vi "MysqlTest2.vi"() -> ()   [LabVIEW 2018]
uses:
  <vilib>/addons/database/Connection.llb/DB Tools Open Connec (String).vi
  <vilib>/addons/database/NI_Database_API.lvlib
panel:
  out "连接的字符串":string
  in  "布尔":bool
  in  "主界面选项卡":enum32{"数据管理"}(tab)
  in  "查询":bool
  in  "终结时间":timestamp
  in  "起始时间":timestamp
  in  "关键字查询":string
  in  "刷新":bool
  out "当前页数":i16
  out "总页数":i16
  in  "下一页":bool
  in  "上一页":bool
  out "数据查询":string[][](table)
  out "data":string[][](table)
  out "error out":errorcluster caption="错误输出"
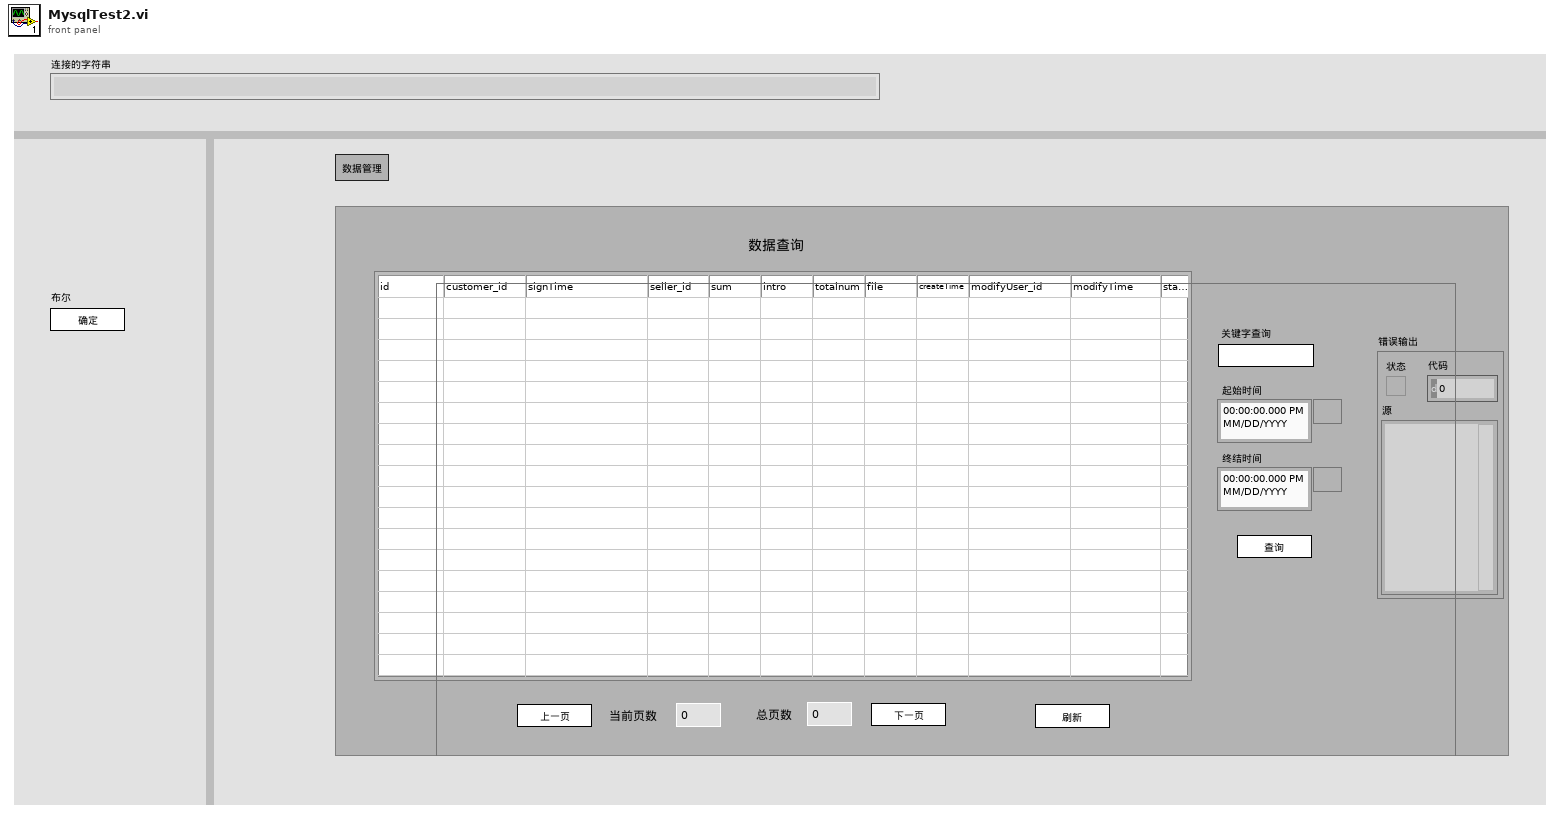
[diagram p1: front panel]
types:
  T1 = typedef "NI_Database_API.lvlib/Conn ObjectReference.ctl" = refnum<k1>
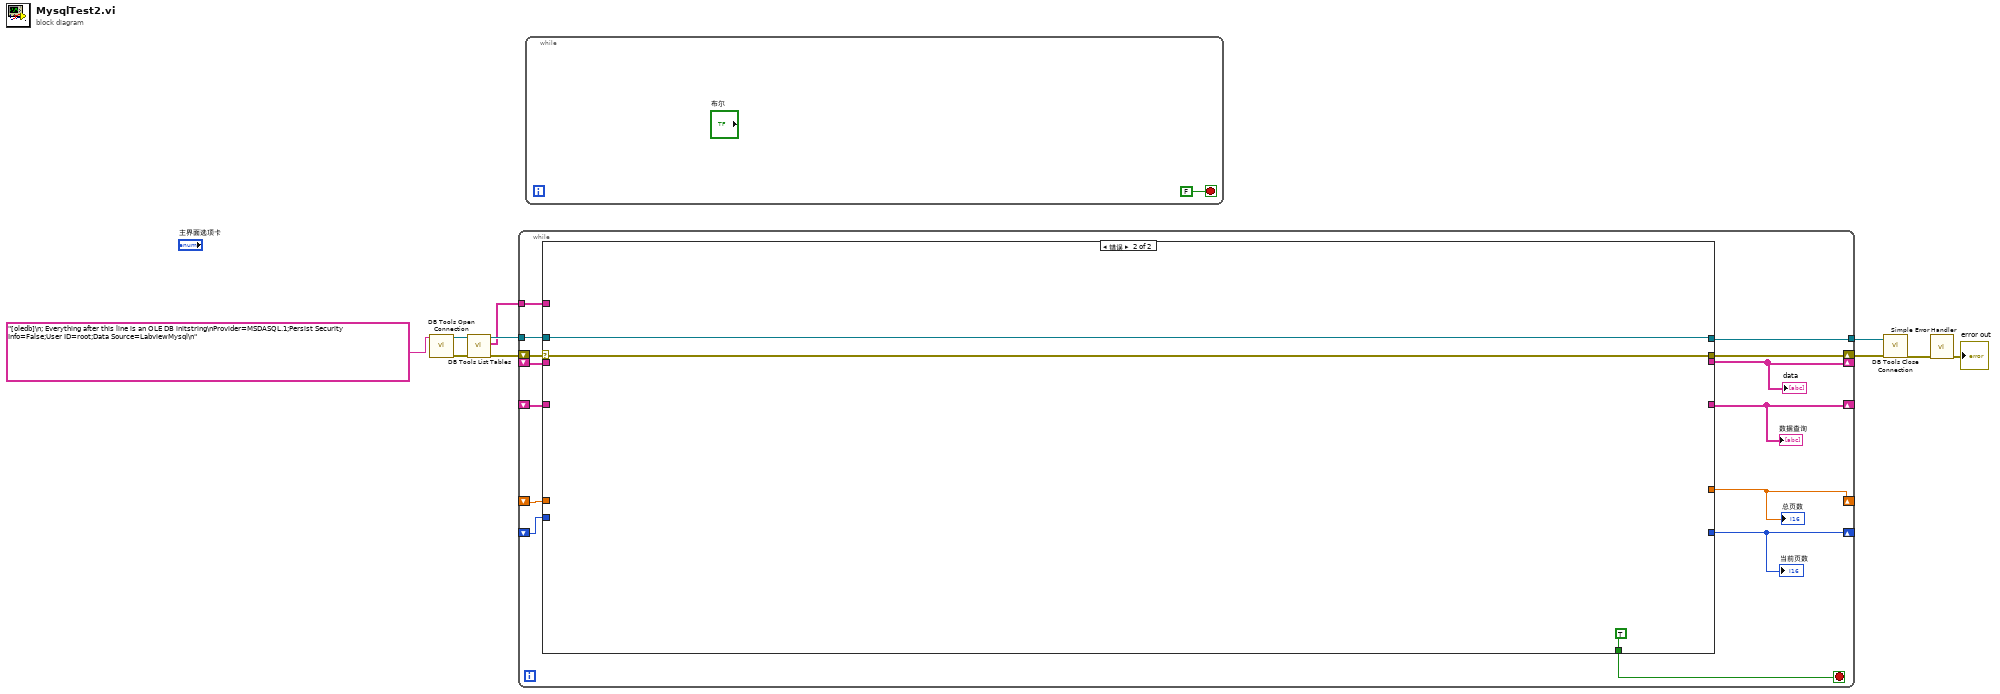
[diagram p0: block diagram]
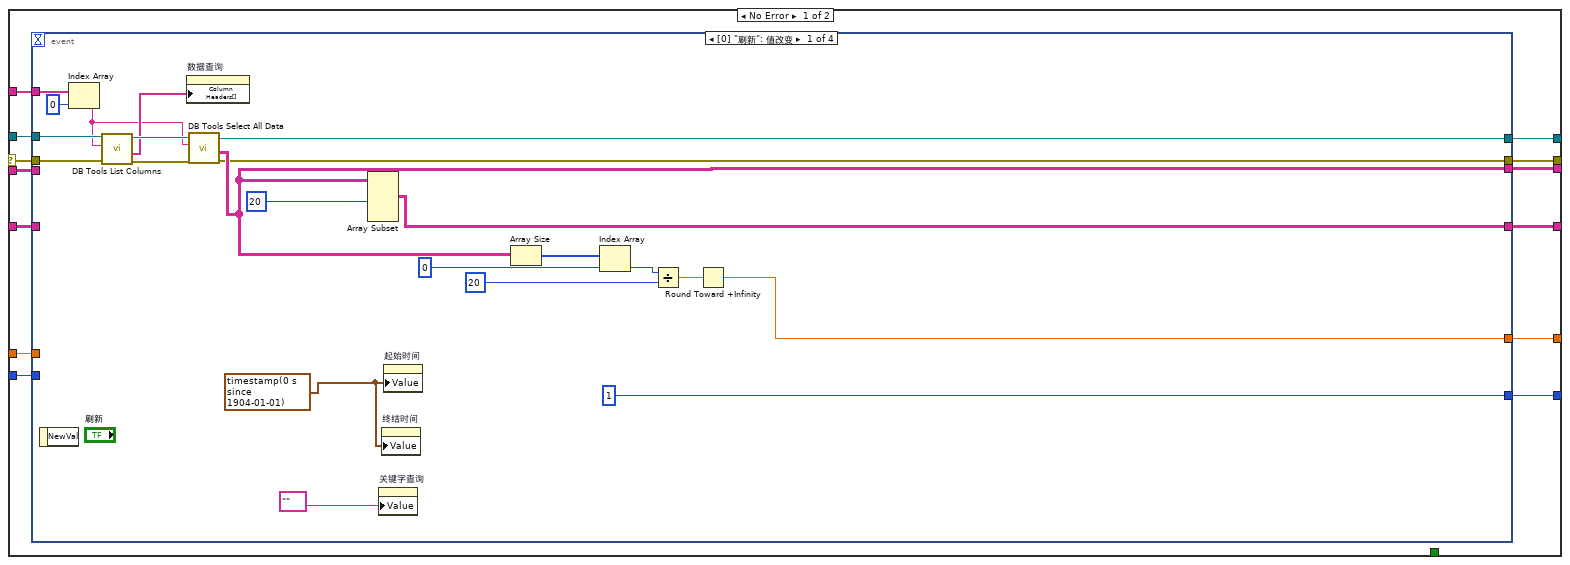
[diagram p2: hidden frame]
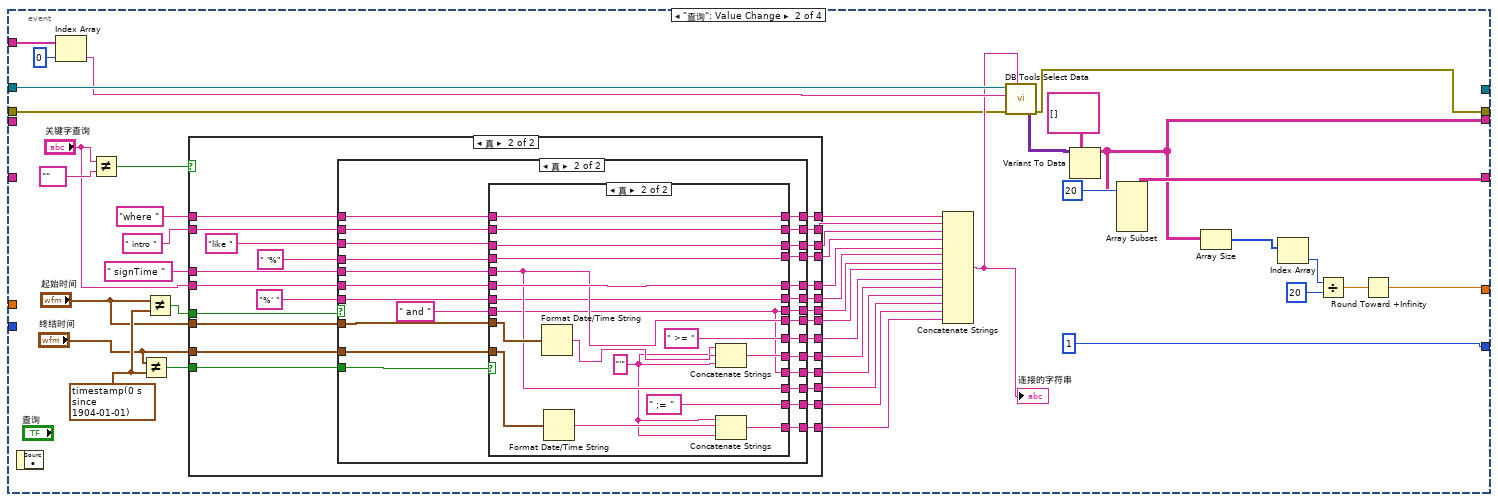
[diagram p3: hidden frame]
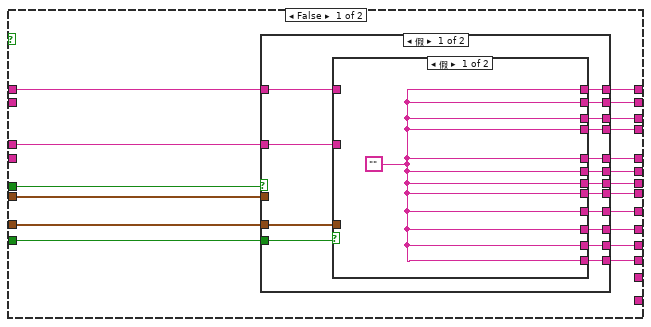
[diagram p4: hidden frame]
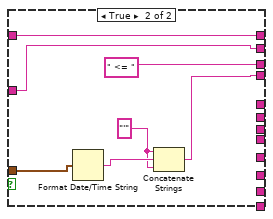
[diagram p5: hidden frame]
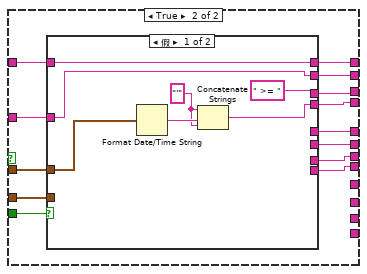
[diagram p6: hidden frame]
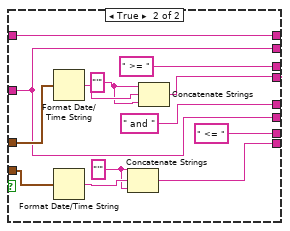
[diagram p7: hidden frame]
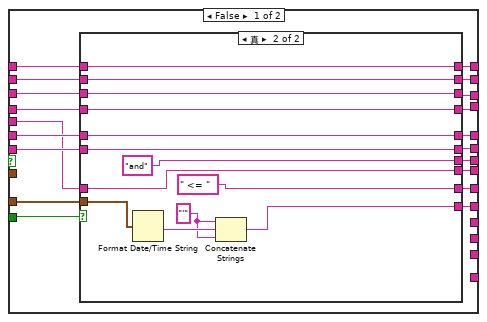
[diagram p8: hidden frame]
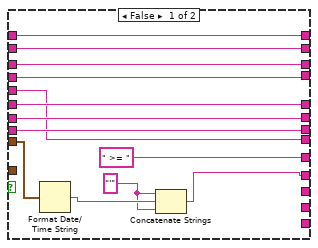
[diagram p10: hidden frame]
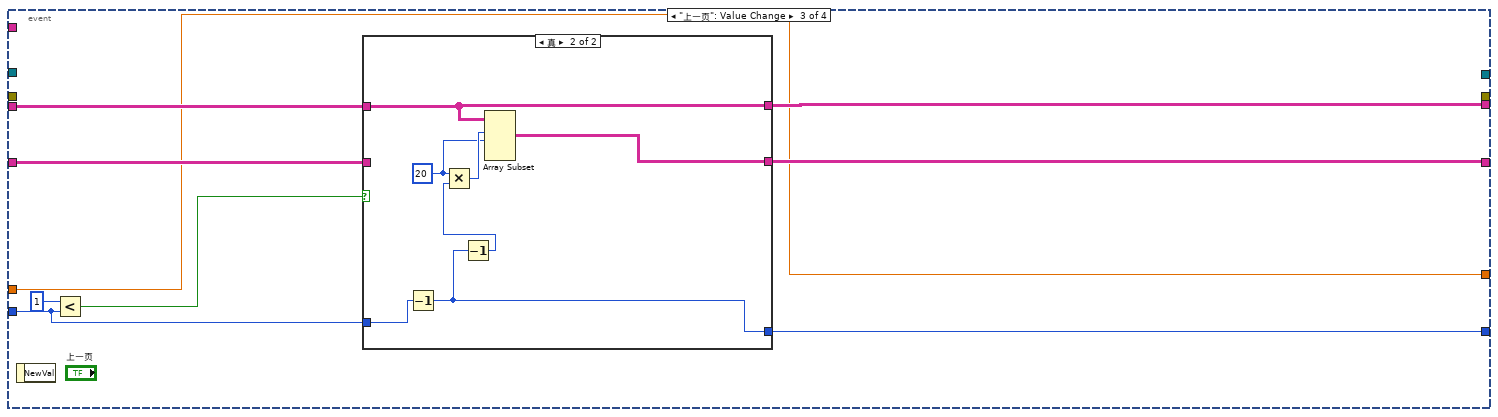
[diagram p11: hidden frame]
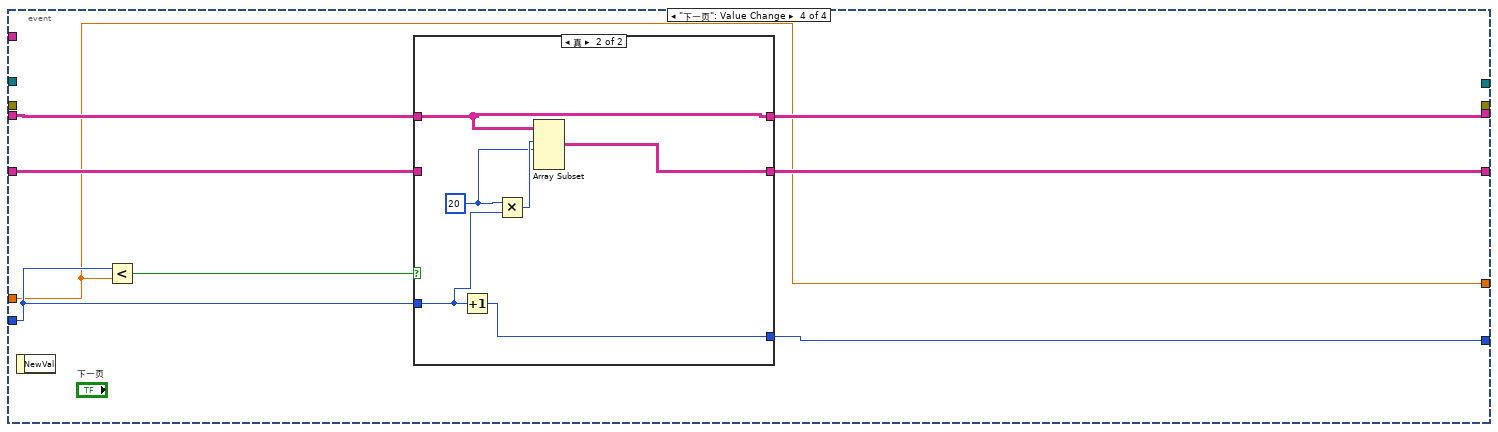
[diagram p13: hidden frame]
diagram:
  n1 = call-poly <vilib>:"DB Tools Open Connection.vi"("connection information"="[oledb]\n; Everything after this line is an OLE DB initstring\nProvider=MSDASQL.1;Persist Security Info=False;User ID=root;Data Source=LabviewMysql\n") -> ("error out"=w5:errorcluster, "connection reference"=w9:T1)  [unwired: 7 in]
  n2 = call <vilib>:"DB Tools List Tables.vi"("error in (no error)"=w5, "connection reference"=w9) -> ("error out"=w4:errorcluster, "tables"=w6:string[], "connection reference out"=w8:T1)  [unwired: 3 in]
  n3 = while {
    tunnel: w8 -> [w24]
    tunnel: [w23] -> w7
    tunnel: w6 -> [w22]
    shift-right: [w21] -> _
    shift-left: _ -> [w19]
    shift-right: [w20] -> _
    shift-left: _ -> [w16]
    shift-right: [w17] -> _
    shift-left: _ -> [w18]
    shift-right: [w15] -> _
    shift-left: _ -> [w14]
    shift-right: [w12] -> w3
    shift-left: w4 -> [w13]
    stop <- w11 stop-if-true
    n4 = case shown="错误" w13 {
      selector: w13 -> [w26 w333]
      tunnel: w24 -> [w37 w334]
      tunnel: [w36 w334] -> w23
      tunnel: w22 -> [w35 _]
      tunnel: [w34 _] -> w21
      tunnel: [w33 _] -> w20
      tunnel: w19 -> [w32 _]
      tunnel: w18 -> [w31 _]
      tunnel: [w30 _] -> w17
      tunnel: w16 -> [w29 _]
      tunnel: [w28 _] -> w15
      tunnel: w14 -> [w27 _]
      tunnel: [w25 w333] -> w12
      tunnel: [_ TRUE] -> w11
      frame No Error {
        n5 = event shown="[0] \"刷新\": 值改变" {
          selector: _ -> [_ _ _ _]
          dyn-events: _ -> [_ _ _ _]
          timeout: _ -> [_ _ _ _]
          tunnel: w37 -> [w59 w100 _ _]
          tunnel: [w55 _ _ _] -> w36
          tunnel: w35 -> [w54 w101 _ _]
          tunnel: [1 1 w300 w316] -> w34
          tunnel: [w45 w63 w296 w315] -> w33
          tunnel: w32 -> [_ _ w302 w317]
          tunnel: [w39 w62 w298 w318] -> w30
          tunnel: w31 -> [_ _ w301 w321]
          tunnel: w29 -> [_ _ w296 w315]
          tunnel: [w44 w68 w299 w320] -> w28
          tunnel: w27 -> [_ _ w297 w319]
          tunnel: w26 -> [w41 w61 _ _]
          tunnel: [w38 w60 _ _] -> w25
          event "刷新": Value Change {
            w42 = timestamp(0 s since 1904-01-01)
            n6 = event-data() -> ()  [unwired: 1 in, 1 out]
            n7 = Index Array(array=w54, index=0 ("索引")) -> (element=w52:string)
            n8 = call <vilib>:"DB Tools List Columns.vi"("error in (no error)"=w41, "table"=w52, "connection reference"=w59) -> ("error out"=w40:errorcluster, "columns"=w56:string[], "connection reference out"=w58:T1)  [unwired: 1 in, 1 out]
            n9 = property on="数据查询" class="Tbl (严格)"("Column Headers[]"=w56) -> ()  [unwired: 2 in, 2 out]
            n10 = call <vilib>:"DB Tools Select All Data.vi"("error in (no error)"=w40, "table"=w52, "connection reference"=w58) -> ("error out"=w38:errorcluster, "data"=w39:string[][], "connection reference out"=w55:T1)  [unwired: 3 in]
            n11 = Array Subset(array=w39, length (row)=20 ("长度")) -> (w44:string[][])  [unwired: 3 in]
            n12 = property on="关键字查询" class="Str"("Value"="") -> ()  [unwired: 2 in, 2 out]
            n13 = property on="终结时间" class="AbsTime (严格)"("Value"=w42) -> ()  [unwired: 2 in, 2 out]
            n14 = property on="起始时间" class="AbsTime (严格)"("Value"=w42) -> ()  [unwired: 2 in, 2 out]
            n15 = Array Size(array=w39) -> (size(s)=w50:i32[])
            n16 = Index Array(array=w50, index=0 ("索引")) -> (element=w48:i32)
            n17 = Divide(x=w48, y=20) -> (x/y=w46:dbl)
            n18 = Round Toward +Infinity(x=w46) -> (ceil(x): smallest int >= x=w45:dbl)
          }
          event "查询": Value Change {
            w97 = timestamp(0 s since 1904-01-01)
            n19 = event-data() -> ()  [unwired: 1 in, 1 out]
            n20 = Index Array(array=w101, index=0 ("索引")) -> (element=w99:string)
            n21 = Not Equal?(x="关键字查询", y="") -> (x != y?=w96:bool)
            n22 = Not Equal?(x="终结时间", y=w97) -> (x != y?=w95:bool)
            n23 = Not Equal?(x="起始时间", y=w97) -> (x != y?=w94:bool)
            n24 = case shown="真" w96 {
              tunnel: w95 -> [w106 w202]
              tunnel: w94 -> [w107 w201]
              tunnel: "where " -> [w108 w200]
              tunnel: " intro " -> [_ w198]
              tunnel: [w120 w199] -> w90
              tunnel: [w119 w197] -> w89
              tunnel: [w118 w196] -> w88
              tunnel: [w117 w195] -> w87
              tunnel: "关键字查询" -> [_ w194]
              tunnel: [w116 w193] -> w86
              tunnel: [w115 w192] -> w85
              tunnel: [w114 w191] -> w84
              tunnel: " signTime " -> [w105 w190]
              tunnel: "起始时间" -> [w103 w189]
              tunnel: "终结时间" -> [w104 w188]
              tunnel: [w113 w187] -> w79
              tunnel: [w112 w186] -> w80
              tunnel: [w111 w185] -> w77
              tunnel: [w110 w184] -> w78
              tunnel: [w109 w183] -> w76
              tunnel: [_ w182] -> w75
              tunnel: [_ w181] -> w74
              frame False {
                n25 = case shown="假" w107 {
                  tunnel: [w136 w156] -> w120
                  tunnel: [w135 w154] -> w119
                  tunnel: [w134 w152] -> w118
                  tunnel: [w133 w151] -> w117
                  tunnel: [w132 w150] -> w116
                  tunnel: [w131 w148] -> w115
                  tunnel: [w130 w147] -> w114
                  tunnel: [w129 w145] -> w113
                  tunnel: [w128 _] -> w112
                  tunnel: [w127 _] -> w111
                  tunnel: [w126 _] -> w110
                  tunnel: [w125 _] -> w109
                  tunnel: w108 -> [w124 w157]
                  tunnel: w106 -> [w123 w155]
                  tunnel: w105 -> [w122 w153]
                  tunnel: w104 -> [w121 w146]
                  tunnel: w103 -> [_ w149]
                  frame False {
                    n26 = case shown="假" w123 {
                      tunnel: [w137 w144] -> w136
                      tunnel: [w137 w143] -> w135
                      tunnel: [w137 " <= "] -> w134
                      tunnel: [w137 w138] -> w133
                      tunnel: [w137 _] -> w132
                      tunnel: [w137 _] -> w131
                      tunnel: [w137 _] -> w130
                      tunnel: [w137 _] -> w129
                      tunnel: [w137 _] -> w128
                      tunnel: [w137 _] -> w127
                      tunnel: [w137 _] -> w126
                      tunnel: [w137 _] -> w125
                      tunnel: w124 -> [_ w144]
                      tunnel: w122 -> [_ w143]
                      tunnel: w121 -> [_ w141]
                      frame False {
                        w137 = ""
                      }
                      frame True {
                        w139 = "'"
                        n27 = Format Date/Time String(seconds (now)=w141) -> (date/time string=w140:string)  [unwired: 2 in]
                        n28 = Concatenate Strings(w139, w140, w139) -> (w138:string)
                      }
                    }
                  }
                  frame True {
                    n29 = case shown="假" w155 {
                      tunnel: w157 -> [w164 w177]
                      tunnel: [w164 w177] -> w156
                      tunnel: [w163 w170] -> w154
                      tunnel: w153 -> [w163 w170]
                      tunnel: [" >= " " >= "] -> w152
                      tunnel: [w158 w172] -> w151
                      tunnel: [_ " and "] -> w150
                      tunnel: w149 -> [w161 w175]
                      tunnel: [_ w170] -> w148
                      tunnel: [_ " <= "] -> w147
                      tunnel: w146 -> [_ w168]
                      tunnel: [_ w165] -> w145
                      frame False {
                        w159 = "'"
                        n30 = Format Date/Time String(seconds (now)=w161) -> (date/time string=w160:string)  [unwired: 2 in]
                        n31 = Concatenate Strings(w159, w160, w159) -> (w158:string)
                      }
                      frame True {
                        w166 = "'"
                        w173 = "'"
                        n32 = Format Date/Time String(seconds (now)=w175) -> (date/time string=w174:string)  [unwired: 2 in]
                        n33 = Format Date/Time String(seconds (now)=w168) -> (date/time string=w167:string)  [unwired: 2 in]
                        n34 = Concatenate Strings(w166, w167, w166) -> (w165:string)
                        n35 = Concatenate Strings(w173, w174, w173) -> (w172:string)
                      }
                    }
                  }
                }
              }
              frame True {
                n36 = case shown="真" w201 {
                  tunnel: w202 -> [w211 w265]
                  tunnel: w200 -> [w221 w264]
                  tunnel: [w220 w263] -> w199
                  tunnel: w198 -> [w219 w262]
                  tunnel: [w218 w261] -> w197
                  tunnel: [w216 w260] -> w196
                  tunnel: [w214 w259] -> w195
                  tunnel: w194 -> [w213 w258]
                  tunnel: [w212 w257] -> w193
                  tunnel: [w209 w256] -> w192
                  tunnel: [w208 w255] -> w191
                  tunnel: w190 -> [w207 w254]
                  tunnel: w189 -> [_ w253]
                  tunnel: w188 -> [w204 w252]
                  tunnel: [w206 w251] -> w187
                  tunnel: [w205 w250] -> w186
                  tunnel: [_ w249] -> w185
                  tunnel: [w203 w248] -> w184
                  tunnel: [_ w247] -> w183
                  tunnel: [_ w246] -> w182
                  tunnel: [_ w245] -> w181
                  tunnel: "like " -> [w217 w244]
                  tunnel: " '%" -> [w215 w243]
                  tunnel: "%' " -> [w210 w242]
                  frame False {
                    n37 = case shown="真" w211 {
                      tunnel: w221 -> [w227 w240]
                      tunnel: [w227 w240] -> w220
                      tunnel: w219 -> [w226 w239]
                      tunnel: [w226 w239] -> w218
                      tunnel: [w225 w238] -> w216
                      tunnel: w217 -> [w225 w238]
                      tunnel: [w224 w237] -> w214
                      tunnel: w215 -> [w224 w237]
                      tunnel: w213 -> [w223 w236]
                      tunnel: [w223 w236] -> w212
                      tunnel: [w222 w235] -> w209
                      tunnel: w210 -> [w222 w235]
                      tunnel: [_ "and"] -> w208
                      tunnel: w207 -> [_ w233]
                      tunnel: [_ w233] -> w206
                      tunnel: [_ " <= "] -> w205
                      tunnel: w204 -> [_ w231]
                      tunnel: [_ w228] -> w203
                      frame False {
                      }
                      frame True {
                        w229 = "'"
                        n38 = Format Date/Time String(seconds (now)=w231) -> (date/time string=w230:string)  [unwired: 2 in]
                        n39 = Concatenate Strings(w229, w230, w229) -> (w228:string)
                      }
                    }
                  }
                  frame True {
                    n40 = case shown="真" w265 {
                      tunnel: w264 -> [w278 w295]
                      tunnel: [w278 w295] -> w263
                      tunnel: w262 -> [w277 w294]
                      tunnel: [w277 w294] -> w261
                      tunnel: [w276 w282] -> w260
                      tunnel: [w275 w281] -> w259
                      tunnel: w258 -> [w274 w293]
                      tunnel: [w274 w293] -> w257
                      tunnel: [w273 w280] -> w256
                      tunnel: [w272 w279] -> w255
                      tunnel: w254 -> [w271 w287]
                      tunnel: w253 -> [w267 w291]
                      tunnel: w252 -> [_ w290]
                      tunnel: [w271 w287] -> w251
                      tunnel: [" >= " " >= "] -> w250
                      tunnel: [_ w279] -> w249
                      tunnel: [w266 w288] -> w248
                      tunnel: [_ w287] -> w247
                      tunnel: [_ " ;= "] -> w246
                      tunnel: [_ w283] -> w245
                      tunnel: w244 -> [w276 w282]
                      tunnel: w243 -> [w275 w281]
                      tunnel: w242 -> [w273 w280]
                      tunnel: " and " -> [w272 w279]
                      frame False {
                        w268 = "'" ("字符串")
                        n41 = Format Date/Time String(seconds (now)=w267) -> (date/time string=w269:string)  [unwired: 2 in]
                        n42 = Concatenate Strings(w268, w269, w268) -> (w266:string)
                      }
                      frame True {
                        w284 = "'"
                        n43 = Format Date/Time String(seconds (now)=w291) -> (date/time string=w289:string)  [unwired: 2 in]
                        n44 = Format Date/Time String(seconds (now)=w290) -> (date/time string=w285:string)  [unwired: 2 in]
                        n45 = Concatenate Strings(w284, w289, w284) -> (w288:string)
                        n46 = Concatenate Strings(w284, w285, w284) -> (w283:string)
                      }
                    }
                  }
                }
              }
            }
            n47 = Concatenate Strings(w90, w89, w88, w87, w86, w85, w84, w79, w80, w78, w77, w76, w75, w74) -> (w73:string)
            "连接的字符串" <- w73
            n48 = call <vilib>:"DB Tools Select Data.vi"("condition"=w73, "error in (no error)"=w61, "table"=w99, "connection reference"=w100) -> ("error out"=w60:errorcluster, "data"=w72:variant[][])  [unwired: 2 in, 1 out]
            n49 = Variant To Data(type=string[][] [], Variant=w72) -> (data=w62:string[][])  [unwired: 1 in, 1 out]
            n50 = Array Subset(array=w62, length (row)=20 ("长度")) -> (w68:string[][])  [unwired: 3 in]
            n51 = Array Size(array=w62) -> (size(s)=w67:i32[])
            n52 = Index Array(array=w67) -> (element=w65:i32)  [unwired: 1 in]
            n53 = Divide(x=w65, y=20) -> (x/y=w66:dbl)
            n54 = Round Toward +Infinity(x=w66) -> (ceil(x): smallest int >= x=w63:dbl)
          }
          event "上一页": Value Change {
            n55 = event-data() -> ()  [unwired: 1 in, 1 out]
            n56 = Less?(x=1, y=w302) -> (x < y?=w303:bool)
            n57 = case shown="真" w303 {
              tunnel: w302 -> [w307 w314]
              tunnel: w301 -> [w306 w310]
              tunnel: [w305 w313] -> w299
              tunnel: [w307 w309] -> w300
              tunnel: [w306 w310] -> w298
              tunnel: w297 -> [w305 _]
              frame False {
              }
              frame True {
                w311 = 20 ("x")
                n58 = Decrement(x=w314) -> (x-1=w309:i32)
                n59 = Decrement(x=w309) -> (x-1=w308:i32)
                n60 = Multiply(x=w311, y=w308) -> (x*y=w312:i32)
                n61 = Array Subset(array=w310, index (row)=w312, length (row)=w311) -> (w313:string[][])  [unwired: 2 in]
              }
            }
          }
          event "下一页": Value Change {
            n62 = event-data() -> ()  [unwired: 1 in, 1 out]
            n63 = Less?(x=w317, y=w315) -> (x < y?=w322:bool)
            n64 = case shown="真" w322 {
              tunnel: w321 -> [w324 w330]
              tunnel: [w325 w331] -> w320
              tunnel: w319 -> [w325 _]
              tunnel: [w324 w330] -> w318
              tunnel: w317 -> [w323 w326]
              tunnel: [w323 w329] -> w316
              frame False {
              }
              frame True {
                w327 = 20 ("x")
                n65 = Increment(x=w326) -> (x+1=w329:i32)
                n66 = Multiply(x=w327, y=w326) -> (x*y=w328:i32)
                n67 = Array Subset(array=w330, index (row)=w328, length (row)=w327) -> (w331:string[][])  [unwired: 2 in]
              }
            }
          }
        }
      }
      frame Error {
      }
    }
    "当前页数" <- w21
    "总页数" <- w20
    "data" <- w17
    "数据查询" <- w15
  }
  n68 = while {
    stop <- FALSE stop-if-true
  }
  n69 = call <vilib>:"DB Tools Close Connection.vi"("error in (no error)"=w3, "connection reference"=w7) -> ("error out"=w2:errorcluster)  [unwired: 5 in]
  n70 = call <vilib>:"Simple Error Handler.vi"("error in (no error)"=w2) -> ("error out"=→"error out":errorcluster)  [unwired: 4 in, 4 out]
